vi "Diode Server.vi"() -> ()   [LabVIEW 2025]
uses:
  <vilib>/addons/_JKI Toolkits/State Machine/_JKI_lib_State_Machine.llb/Select State(s)_err__jki_lib_state_machine.vi
  <vilib>/addons/_JKI Toolkits/State Machine/_JKI_lib_State_Machine.llb/Periodic Trigger__ogtk__JKI-SM__jki_lib_state_machine.vi
  <instrlib>/ULx/ULx_LV.dll
  <instrlib>/Keithley 648X Series/Keithley 648X Series.lvlib
  <userlib>/_OpenG.lib/comparison/comparison.llb/openg_comparison__ogtk.lvlib
  <userlib>/_OpenG.lib/comparison/comparison.llb/Boolean Changed__ogtk.vi
panel:
  in  "Stimulate_LED":refnum<k21>
  in  "LED_Stimulate":bool
  in  "LED_Illuminate":bool
  out "D0 Measurement":dbl
  out "D1 Measurement":dbl
  in  "Illuminate_LED":refnum<k21>
  in  "MWIR PicoAmmeter":refnum<visa-resource-name>
  in  "SWIR Input":refnum<k21>="Dev0/Ai0"
  out "Diode Currents":waveform(dbl)[](graph)
  in  "Exit":bool
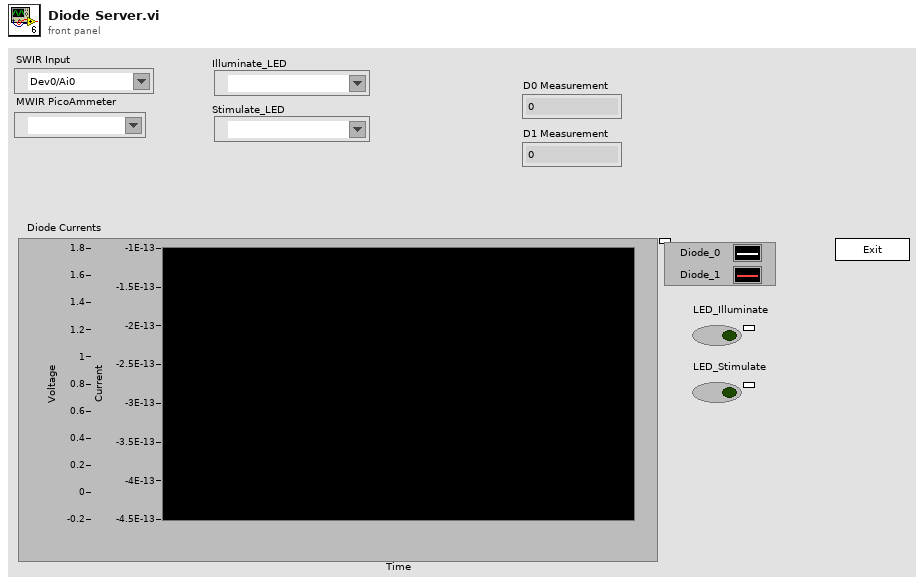
[diagram p1: front panel]
types:
  T1 = enum32{"Invalid", "Standard", "Closed", "Hidden", "Minimized", "Maximized"}
  T2 = enum32{"invalid app kind", "Development System", "Run Time System", "Student Edition", "Embedded LabVIEW", "Evaluation", "Custom"}
  T3 = cluster{"Core":cluster{"Current VI Reference":refnum<vi>, "Close Panel on Exit?":bool}, "Diode_Wfm":cluster{"Diode_Wfm":waveform(dbl)[]}, "Ulx SWIRMon":refnum<k24>, "ULx LED_Illum":refnum<k24>, "ULx LED_Stim":refnum<k24>, "PicoAmmeter VISA":refnum<visa-resource-name>}
  T4 = cluster{"Current VI Reference":refnum<vi>, "Close Panel on Exit?":bool}
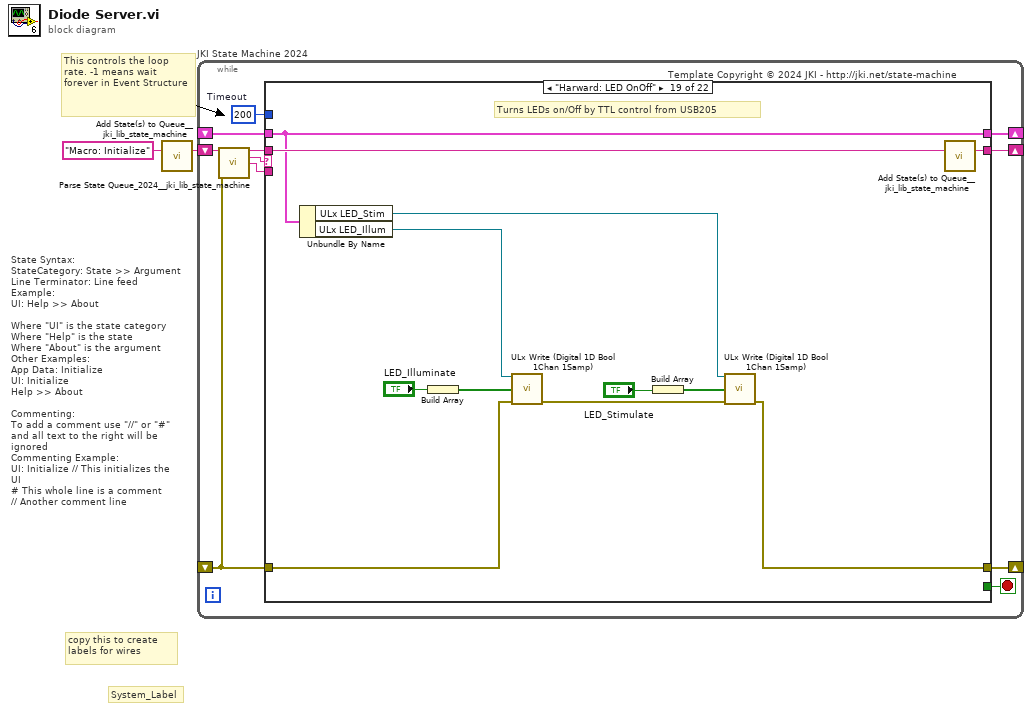
[diagram p0: block diagram]
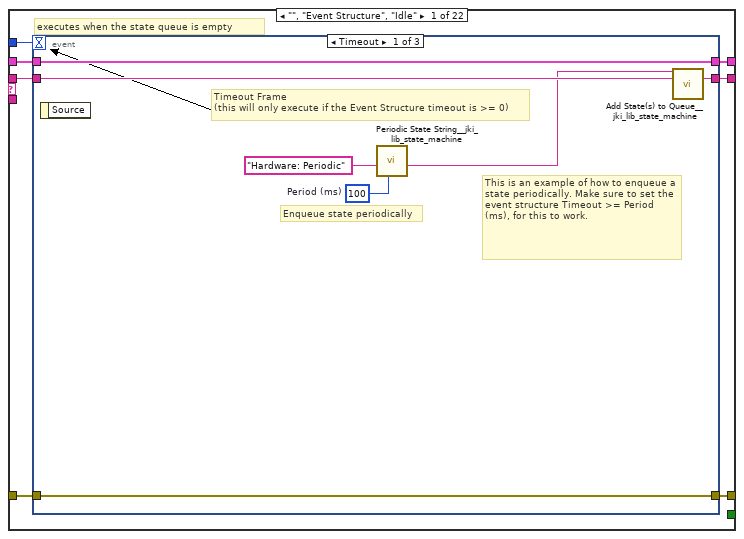
[diagram p2: hidden frame]
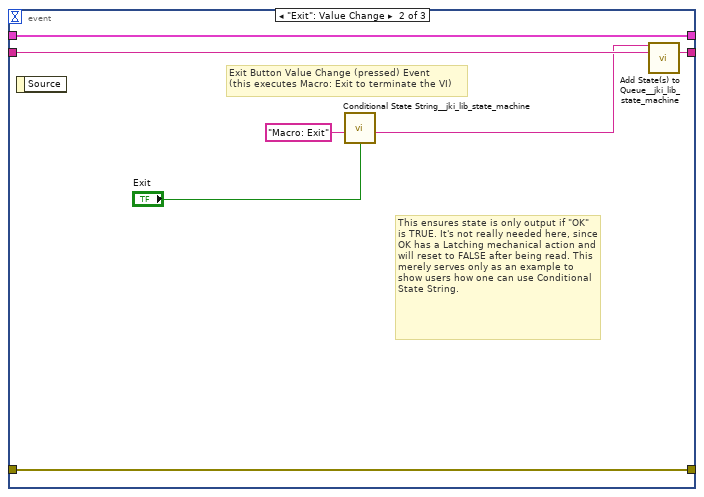
[diagram p3: hidden frame]
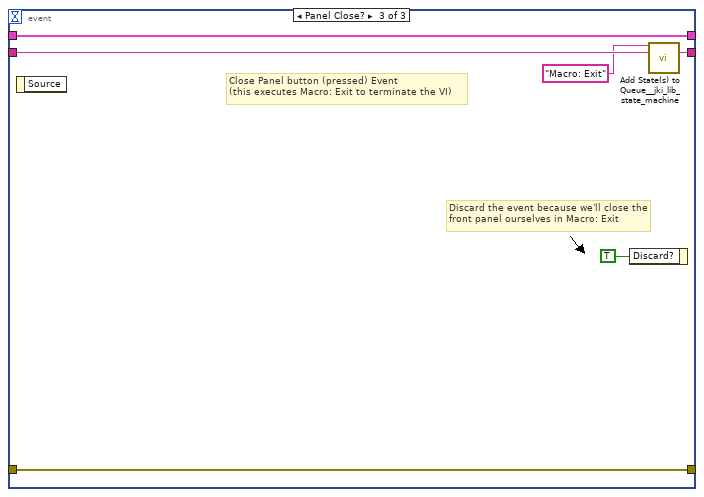
[diagram p4: hidden frame]
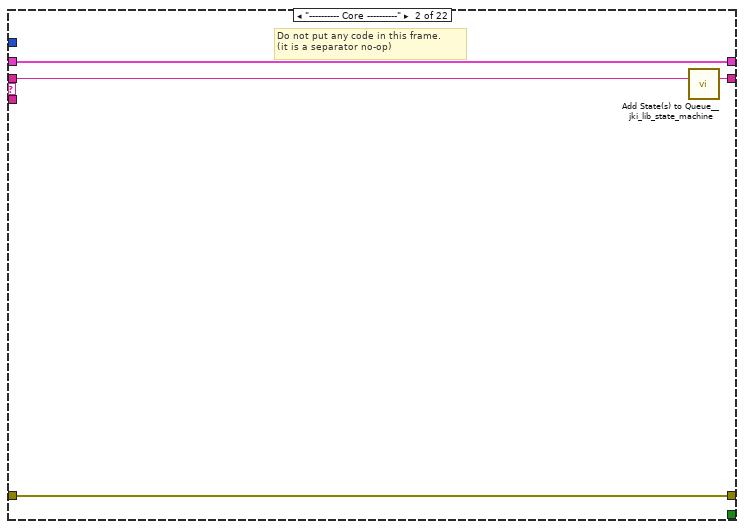
[diagram p5: hidden frame]
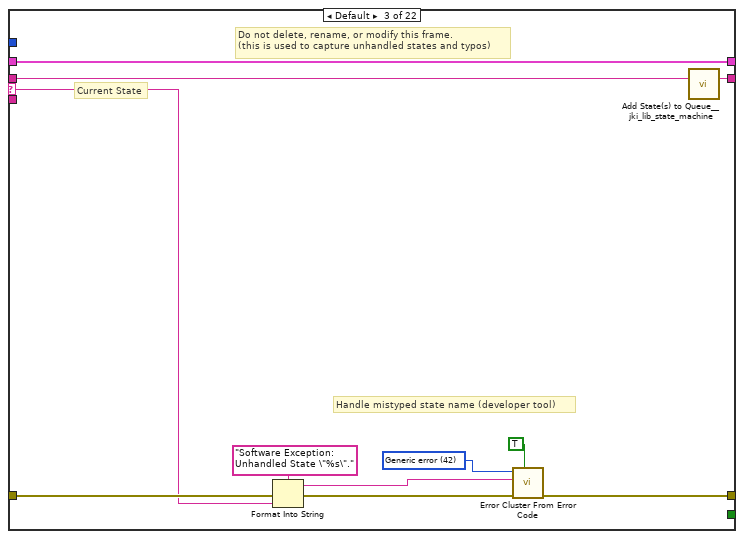
[diagram p6: hidden frame]
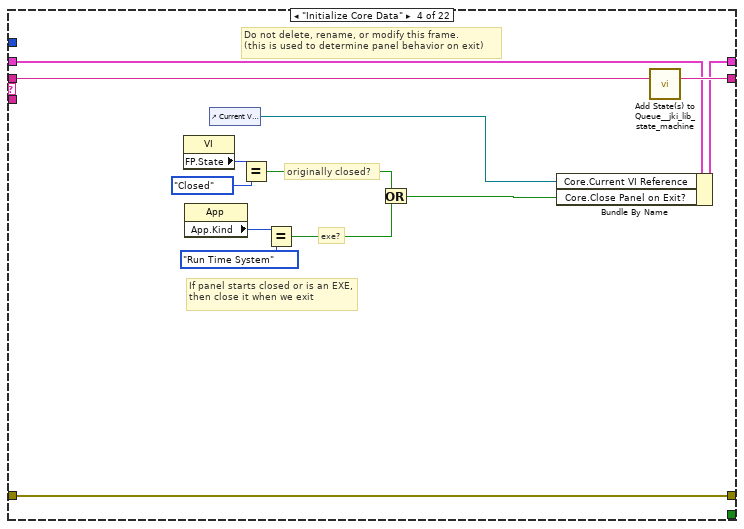
[diagram p7: hidden frame]
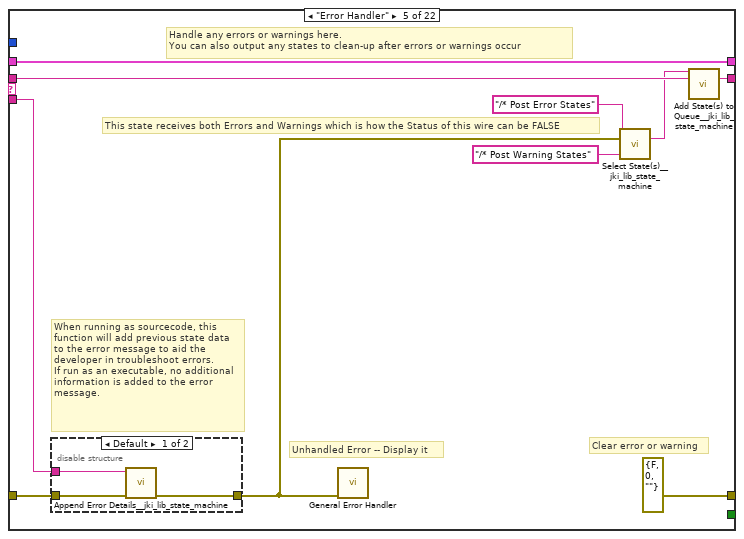
[diagram p8: hidden frame]
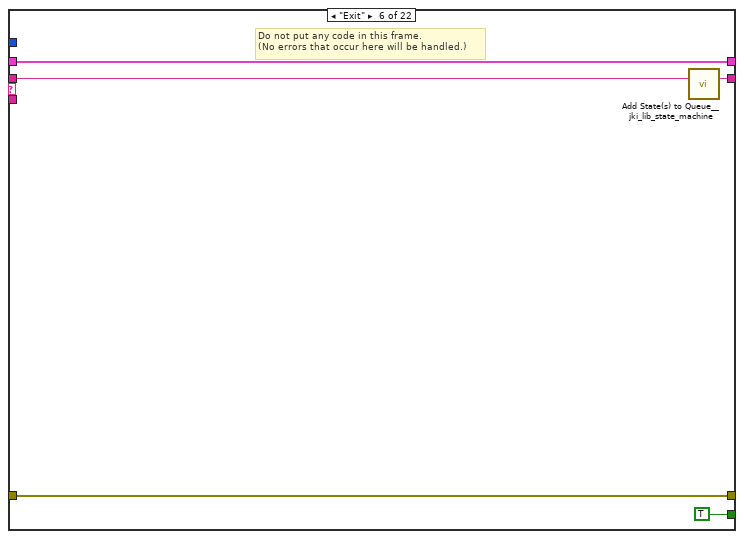
[diagram p10: hidden frame]
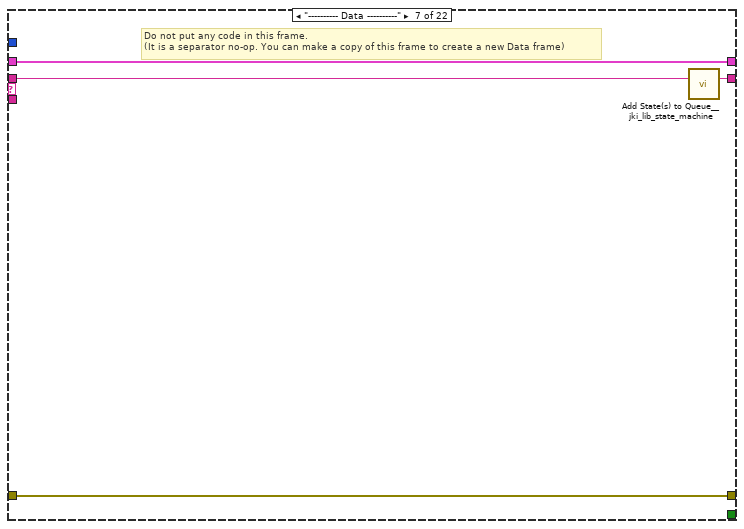
[diagram p11: hidden frame]
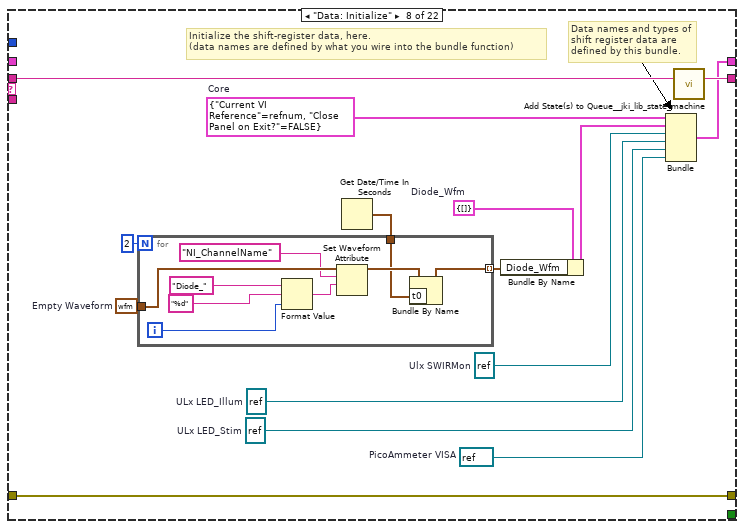
[diagram p12: hidden frame]
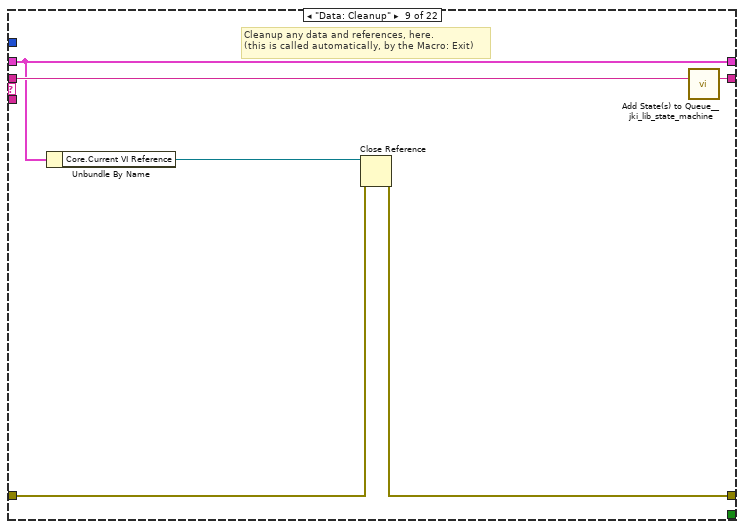
[diagram p13: hidden frame]
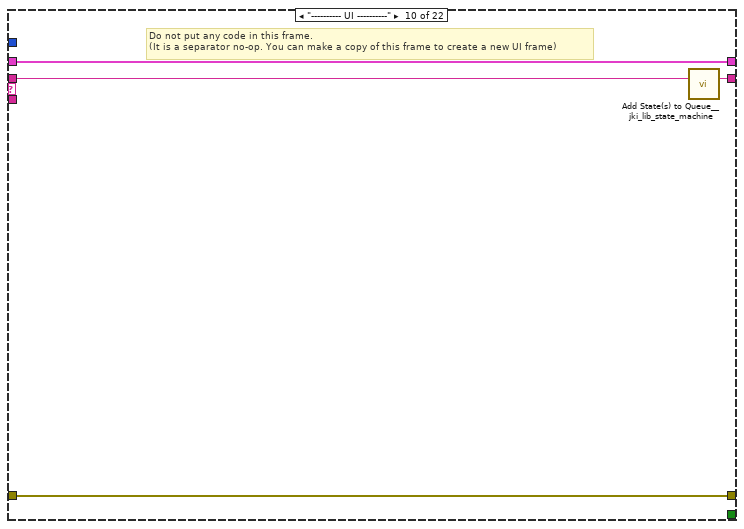
[diagram p14: hidden frame]
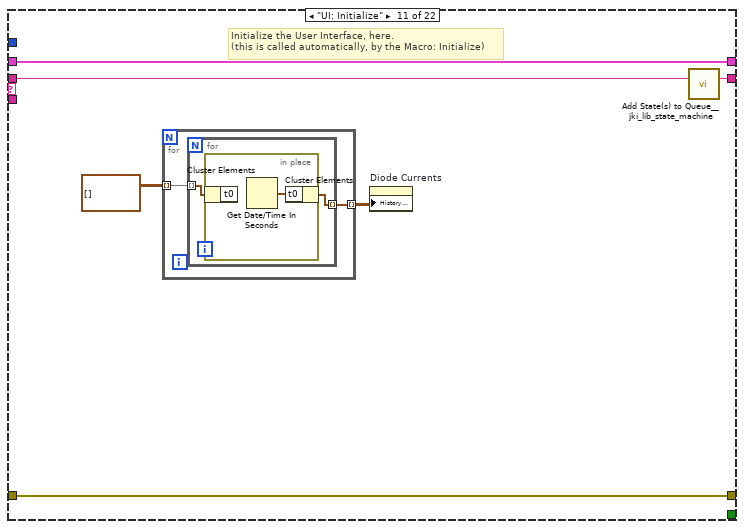
[diagram p15: hidden frame]
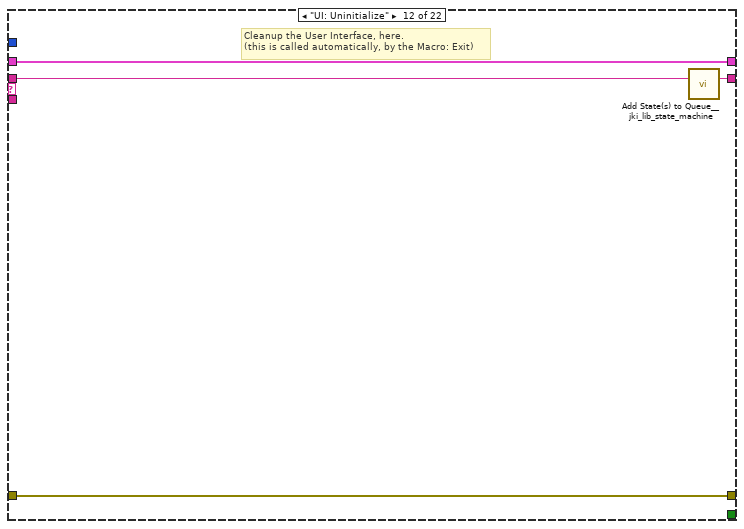
[diagram p16: hidden frame]
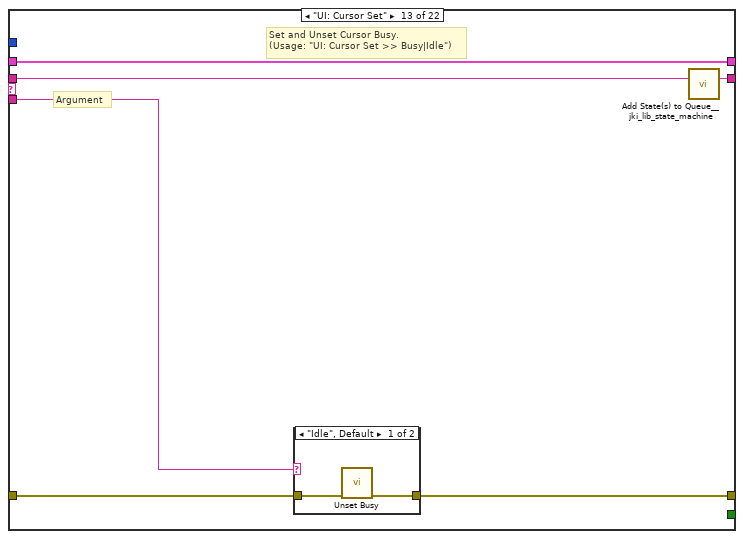
[diagram p17: hidden frame]
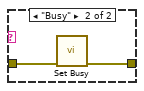
[diagram p18: hidden frame]
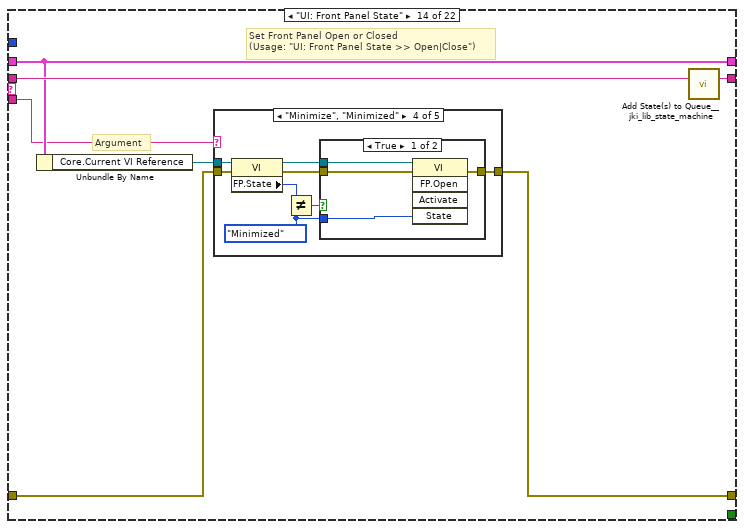
[diagram p19: hidden frame]
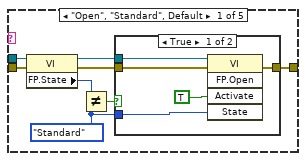
[diagram p20: hidden frame]
diagram:
  # "State Syntax:\nStateCategory: State >> Argument\nLine Terminator: Line feed\nExample:\nUI: Help >> About\n\nWhere \"UI\" is the state category\nWhere \"Help\" is the state\nWhere \"About\" is the argument\nOther Examples:\nApp Data: Initialize\nUI: Initialize\nHelp >> About\n\nCommenting:\nTo add a comment use \"//\" or \"#\" and all text to the right will be ignored\nCommenting Example:\nUI: Initialize // This initializes the UI\n# This whole line is a comment\n// Another comment line"
  # "copy this to create labels for wires"
  # "This controls the loop rate. -1 means wait forever in Event Structure"
  # "System_Label"
  n1 = call <vilib>:"Add State(s) to Queue__jki_lib_state_machine.vi"("State(s) in (\"\")"="Macro: Initialize") -> ("States Out"=w2:string)  [unwired: 14 in]
  n2 = while "JKI State Machine 2024" {
    shift-right: [w6] -> _
    shift-left: _ -> [w5]
    shift-right: [w9] -> _
    shift-left: _ -> [w3]
    shift-right: [w8] -> _
    shift-left: w2 -> [w10]
    stop <- w7 stop-if-true
    w4 = 200  # Timeout
    # "Template Copyright © 2024 JKI - http://jki.net/state-machine"
    n3 = call <vilib>:"Parse State Queue_2024__jki_lib_state_machine.vi"("State Queue"=w10, "Error In (no error)"=w3) -> ("Remaining States"=w12:string, "Current State"=w13:string, "Arguments"=w11:string)  [unwired: 11 in]
    n4 = case shown="\"Harward: LED OnOff\"" w13 {
      selector: w13 -> [_ _ w45 _ _ _ _ _ _ _ _ _ _ _ _ _ _ _ _ _ _ _]
      tunnel: w12 -> [w20 w44 w49 w68 w78 w87 w91 w106 w121 w125 w131 w140 w146 w157 w226 w231 w240 w244 w256 w275 w287 w305]
      tunnel: w11 -> [_ _ _ _ w73 _ _ _ _ _ _ _ w141 w151 _ _ _ _ _ _ _ _]
      tunnel: w5 -> [w18 w41 w47 w61 w75 w85 w88 _ w116 w122 w129 w138 w144 w153 w223 w228 w238 w241 w254 w273 w285 w298]
      tunnel: [w17 w42 w51 w65 errorcluster {"status"=FALSE, "code"=0, "source"=""} ("error out") w84 w89 w103 w117 w123 w128 w137 w142 w154 w224 w229 w235 w242 w247 w266 w281 w301] -> w9
      tunnel: w3 -> [w14 w42 w50 w65 w74 w84 w89 w103 w118 w123 w128 w137 w143 w155 w224 w229 w235 w242 w250 w271 w282 w302]
      tunnel: [w19 w43 w48 w67 w77 w86 w90 w105 w120 w124 w130 w139 w145 w156 w225 w230 w239 w243 w255 w274 w286 w304] -> w8
      tunnel: [_ _ _ _ _ TRUE _ _ _ _ _ _ _ _ _ _ _ _ _ _ _ _] -> w7
      tunnel: [w16 w41 w47 w66 w75 w85 w88 w104 w116 w122 w129 w138 w144 w153 w223 w228 w238 w241 w254 w268 w285 w296] -> w6
      tunnel: w4 -> [w15 _ _ _ _ _ _ _ _ _ _ _ _ _ _ _ _ _ _ _ _ _]
      frame "", "Event Structure", "Idle" {
        # "executes when the state queue is empty"
        n5 = event shown="[0] Timeout" {
          selector: _ -> [_ _ _]
          dyn-events: _ -> [_ _ _]
          timeout: w15 -> [_ _ _]
          tunnel: w20 -> [w27 w34 w40]
          tunnel: [w26 w33 w39] -> w19
          tunnel: w18 -> [w24 w31 w37]
          tunnel: [w25 w32 w38] -> w17
          tunnel: w14 -> [w25 w32 w38]
          tunnel: [w24 w31 w37] -> w16
          event Timeout {
            w21 = u32 100  # Period (ms)
            # "Enqueue state periodically"
            # "This is an example of how to enqueue a state periodically. Make sure to set the event structure Timeout >= Period (ms), for this to work."
            # "Timeout Frame\n(this will only execute if the Event Structure timeout is >= 0)"
            n6 = event-data() -> ()  [unwired: 1 in, 1 out]
            n7 = call <vilib>:"Periodic State String__jki_lib_state_machine.vi"("Period (ms)"=w21, "State"="Hardware: Periodic") -> ("State Out"=w23:string)  [unwired: 9 in]
            n8 = call <vilib>:"Add State(s) to Queue__jki_lib_state_machine.vi"("State(s) in Front (\"\")"=w23, "State(s) in (\"\")"=w27) -> ("States Out"=w26:string)  [unwired: 13 in]
          }
          event "Exit": Value Change {
            # "This ensures state is only output if \"OK\" is TRUE. It's not really needed here, since OK has a Latching mechanical action and will reset to FALSE after being read. This merely serves only as an example to show users how one can use Conditional State String."
            # "Exit Button Value Change (pressed) Event\n(this executes Macro: Exit to terminate the VI)"
            n9 = event-data() -> ()  [unwired: 1 in, 1 out]
            n10 = call <vilib>:"Conditional State String__jki_lib_state_machine.vi"("Do State(s)?"="Exit", "State"="Macro: Exit") -> ("State Out"=w28:string)  [unwired: 7 in]
            n11 = call <vilib>:"Add State(s) to Queue__jki_lib_state_machine.vi"("State(s) in Front (\"\")"=w28, "State(s) in (\"\")"=w34) -> ("States Out"=w33:string)  [unwired: 13 in]
          }
          event Panel Close? {
            # "Discard the event because we'll close the front panel ourselves in Macro: Exit"
            # "Close Panel button (pressed) Event\n(this executes Macro: Exit to terminate the VI)"
            n12 = event-data() -> ()  [unwired: 1 in, 1 out]
            n13 = event-data("Discard?"=TRUE) -> ()  [unwired: 1 in, 1 out]
            n14 = call <vilib>:"Add State(s) to Queue__jki_lib_state_machine.vi"("State(s) in Front (\"\")"="Macro: Exit", "State(s) in (\"\")"=w40) -> ("States Out"=w39:string)  [unwired: 13 in]
          }
        }
      }
      frame "---------- Core ----------" {
        # "Do not put any code in this frame.\n(it is a separator no-op)"
        n15 = call <vilib>:"Add State(s) to Queue__jki_lib_state_machine.vi"("State(s) in (\"\")"=w44) -> ("States Out"=w43:string)  [unwired: 14 in]
      }
      frame Default {
        w54 = 42 items=["No error", "Argument error", "Memory is full", "Out of zone", "End of file", "File already open", "Generic file I/O error", "File not found", "File permission error", "Disk is full", "Duplicate path", "Too many files open", "System feature not enabled", "Resource file not found", "Cannot add resource", "Resource not found", "Image not found", "Image memory error", "Pen does not exist", "Config type invalid", "Config token not found", "Config parse error", "Config memory error", "Bad external code format", "Bad external code offset", "External code not present", "Null window", "Destroy window error", "Null menu", "Print aborted", "Bad print record", "Print driver error", "Windows error during printing", "Memory error during printing", "Print dialog error", "Generic print error", "Invalid device refnum", "Device not found", "Device parameter error", "Device unit error", "Cannot open device", "Device call aborted", "Generic error", "Cancelled by user", "Object ID too low", "Object ID too high", "Object not in heap", "Unknown heap", "Unknown object (invalid DefProc)", "Unknown object (DefProc not in table)", "Message out of range", "Invalid (null) method", "Unknown message", "Manager call not supported", "Bad address", "Network operation in progress", "Network operation timed out", "Connection is busy", "Network attribute not supported", "Network error", "Address in use", "System out of memory", "Connection aborted", "Connection refused", "Not connected", "Already connected", "Connection closed", "Initialization error (interapplication manager)", "Bad occurrence", "Wait on unbound occurrence handler", "Occurrence queue overflow", "Datalog type conflict", "Unused", "Unrecognized type (interapplication manager)", "Memory corrupt", "Failed to make temporary DLL", "Old CIN version", "Drag socket not found", "Failed to load drop-object", "Failed to register OLE object", "Failed to release OLE object", "Format specifier type mismatch", "Unknown format specifier", "Too few format specifiers", "Too many format specifiers", "Scan failed", "Newer CIN version", "Error converting to variant", "Runtime menu error", "Password tampered", "Variant attribute not found", "Incompatible variant data type", "Event data is not available", "Event Store is not present", "Occurrence is not found", "Event Queue is not created", "Event info is not available", "Refnum passed is NULL", "Error retrieving Class GUID", "Error retrieving CoClass GUID", "Error retrieving TypeLib GUID.", "Bad built application magic bytes.", "Specific driver is different from the specific driver associated with the Logical Name.", "There is no session opened to the class driver.", "Max Error", "MAX - Error with config objects", "MAX - Error loading configuration", "MAX - Group not supported"]
        # "Current State"
        # "Do not delete, rename, or modify this frame.\n(this is used to capture unhandled states and typos)"
        # "Handle mistyped state name (developer tool)"
        n16 = Format Into String(format string="Software Exception: Unhandled State \"%s\"." ("message"), error in=w50, w45) -> (resulting string=w53:string, error out=w52:errorcluster)  [unwired: 1 in]
        n17 = call <vilib>:"Error Cluster From Error Code.vi"("show call chain? (False)"=TRUE, "error in (no error)"=w52, "error message (\"\")"=w53, "error code (0)"=w54) -> ("error out"=w51:errorcluster)  [unwired: 5 in]
        n18 = call <vilib>:"Add State(s) to Queue__jki_lib_state_machine.vi"("State(s) in (\"\")"=w49) -> ("States Out"=w48:string)  [unwired: 14 in]
      }
      frame "Initialize Core Data" {
        # "Do not delete, rename, or modify this frame.\n(this is used to determine panel behavior on exit)"
        # "originally closed?"
        # "exe?"
        # "If panel starts closed or is an EXE, then close it when we exit"
        n19 = property class="VI"() -> ("FP.State"=w58:T1)  [unwired: 2 in, 2 out]
        n20 = property class="App"() -> ("App.Kind"=w64:T2)  [unwired: 2 in, 2 out]
        n21 = control-ref of="Current VI Reference"() -> (w59:refnum<vi>)
        n22 = Equal?(x=w58, y=T1."Closed" ("Front Panel Window:State")) -> (x = y?=w56:bool)
        n23 = Equal?(x=w64, y=T2."Run Time System" ("Application:Kind")) -> (x = y?=w62:bool)
        n24 = Or(x=w56, y=w62) -> (x .or. y?=w60:bool)
        n25 = Bundle By Name(cluster=w61, "Core.Current VI Reference"=w59, "Core.Close Panel on Exit?"=w60) -> (w66:T3)
        n26 = call <vilib>:"Add State(s) to Queue__jki_lib_state_machine.vi"("State(s) in (\"\")"=w68) -> ("States Out"=w67:string)  [unwired: 14 in]
      }
      frame "Error Handler" {
        # "When running as sourcecode, this function will add previous state data to the error message to aid the developer in troubleshoot errors.\nIf run as an executable, no additional information is added to the error message."
        # "This state receives both Errors and Warnings which is how the Status of this wire can be FALSE"
        # "Unhandled Error -- Display it"
        # "Handle any errors or warnings here.\nYou can also output any states to clean-up after errors or warnings occur"
        # "Clear error or warning"
        n27 = disable-structure shown="Default" {
          disable-tunnel: w74 -> [w81 w82]
          disable-tunnel: w73 -> [w80 _]
          disable-tunnel: [w79 w82] -> w72
          frame condition #0 (active) {
            n28 = call <vilib>:"Append Error Details__jki_lib_state_machine.vi"("error in (no error)"=w81, "Previous State and Argument(s)"=w80) -> ("error out"=w79:errorcluster)  [unwired: 9 in]
          }
          frame condition #1 {
          }
        }
        n29 = call <vilib>:"General Error Handler.vi"("error in (no error)"=w72) -> ()  [unwired: 10 in, 5 out]
        n30 = call-poly <vilib>:"Select State(s)__jki_lib_state_machine.vi"("State(s) if True (\"\")"="/* Post Error States", "Select"=w72, "State(s) if False (\"\")"="/* Post Warning States") -> ("States Out"=w70:string)  [unwired: 12 in]
        n31 = call <vilib>:"Add State(s) to Queue__jki_lib_state_machine.vi"("State(s) in Front (\"\")"=w70, "State(s) in (\"\")"=w78) -> ("States Out"=w77:string)  [unwired: 13 in]
      }
      frame "Exit" {
        # "Do not put any code in this frame.\n(No errors that occur here will be handled.)"
        n32 = call <vilib>:"Add State(s) to Queue__jki_lib_state_machine.vi"("State(s) in (\"\")"=w87) -> ("States Out"=w86:string)  [unwired: 14 in]
      }
      frame "---------- Data ----------" {
        # "Do not put any code in this frame.\n(It is a separator no-op. You can make a copy of this frame to create a new Data frame)"
        n33 = call <vilib>:"Add State(s) to Queue__jki_lib_state_machine.vi"("State(s) in (\"\")"=w91) -> ("States Out"=w90:string)  [unwired: 14 in]
      }
      frame "Data: Initialize" {
        w92 = refnum<k24> refnum  # ULx LED_Stim
        w100 = cluster{"Diode_Wfm":waveform(dbl)[]} {"Diode_Wfm"=[]}  # Diode_Wfm
        w94 = refnum<visa-resource-name> refnum  # PicoAmmeter VISA
        w93 = refnum<k24> refnum  # ULx LED_Illum
        w96 = refnum<k24> refnum  # Ulx SWIRMon
        w98 = waveform(dbl) {"t0"=timestamp(0 s since 1904-01-01), "dt"=1.0, "Y"=[]}  # Empty Waveform
        w102 = T4 {"Current VI Reference"=refnum, "Close Panel on Exit?"=FALSE}  # Core
        # "Data names and types of shift register data are defined by this bundle."
        # "Initialize the shift-register data, here.\n(data names are defined by what you wire into the bundle function)"
        n34 = Get Date/Time In Seconds() -> (seconds since 1Jan1904=w95:timestamp)
        n35 = for {
          N: 2 -> [_]
          tunnel: w98 -> [w112]
          tunnel: [w108] -> w101 mode=indexing
          tunnel: w95 -> [w107]
          i -> [w109]
          n36 = Format Value(string ("")="Diode_", format string="%d", value (0)=w109) -> (output string=w114:string)
          n37 = Set Waveform Attribute(5:w114, 6:"NI_ChannelName" ("name"), 7:w112) -> (3:w111:waveform(dbl))  [unwired: 1 in, 2 out]
          n38 = Bundle By Name(cluster=w111, "t0"=w107) -> (w108:waveform(dbl))
        }
        n39 = Bundle By Name(cluster=w100, "Diode_Wfm"=w101) -> (w97:cluster{"Diode_Wfm":waveform(dbl)[]})
        n40 = Bundle("Core"=w102, "Diode_Wfm"=w97, "Ulx SWIRMon"=w96, "ULx LED_Illum"=w93, "ULx LED_Stim"=w92, "PicoAmmeter VISA"=w94) -> (w104:T3)  [unwired: 1 in]
        n41 = call <vilib>:"Add State(s) to Queue__jki_lib_state_machine.vi"("State(s) in (\"\")"=w106) -> ("States Out"=w105:string)  [unwired: 14 in]
      }
      frame "Data: Cleanup" {
        # "Cleanup any data and references, here.\n(this is called automatically, by the Macro: Exit)"
        n42 = Unbundle By Name(w116) -> ("Core.Current VI Reference"=w119:refnum<vi>)
        n43 = Close Reference(reference=w119, error in (no error)=w118) -> (error out=w117:errorcluster)
        n44 = call <vilib>:"Add State(s) to Queue__jki_lib_state_machine.vi"("State(s) in (\"\")"=w121) -> ("States Out"=w120:string)  [unwired: 14 in]
      }
      frame "---------- UI ----------" {
        # "Do not put any code in this frame.\n(It is a separator no-op. You can make a copy of this frame to create a new UI frame)"
        n45 = call <vilib>:"Add State(s) to Queue__jki_lib_state_machine.vi"("State(s) in (\"\")"=w125) -> ("States Out"=w124:string)  [unwired: 14 in]
      }
      frame "UI: Initialize" {
        # "Initialize the User Interface, here.\n(this is called automatically, by the Macro: Initialize)"
        n46 = for {
          tunnel: waveform(dbl)[][] [] ("History Data") -> [w133] mode=indexing
          tunnel: [w132] -> w126 mode=indexing
          n47 = for {
            tunnel: w133 -> [w135] mode=indexing
            tunnel: [w134] -> w132 mode=indexing
            n48 = in-place {
              n49 = in-place-cluster #1(w135) -> ()  [unwired: 1 out]
              n50 = Get Date/Time In Seconds() -> (seconds since 1Jan1904=w136:timestamp)
              n51 = in-place-cluster #1("t0"=w136) -> (w134:waveform(dbl))
            }
          }
        }
        n52 = property on="Diode Currents" class="WFChart (strict)"("History Data"=w126) -> ()  [unwired: 2 in, 2 out]
        n53 = call <vilib>:"Add State(s) to Queue__jki_lib_state_machine.vi"("State(s) in (\"\")"=w131) -> ("States Out"=w130:string)  [unwired: 14 in]
      }
      frame "UI: Uninitialize" {
        # "Cleanup the User Interface, here.\n(this is called automatically, by the Macro: Exit)"
        n54 = call <vilib>:"Add State(s) to Queue__jki_lib_state_machine.vi"("State(s) in (\"\")"=w140) -> ("States Out"=w139:string)  [unwired: 14 in]
      }
      frame "UI: Cursor Set" {
        # "Argument"
        # "Set and Unset Cursor Busy.\n(Usage: \"UI: Cursor Set >> Busy|Idle\")"
        n55 = case shown="\"Idle\", Default" w141 {
          tunnel: w143 -> [w148 w150]
          tunnel: [w147 w149] -> w142
          frame "Idle", Default {
            n56 = call <vilib>:"Unset Busy.vi"("error in (no error)"=w148) -> ("error out"=w147:errorcluster)  [unwired: 10 in]
          }
          frame "Busy" {
            n57 = call <vilib>:"Set Busy.vi"("error in (no error)"=w150) -> ("error out"=w149:errorcluster)  [unwired: 9 in, 1 out]
          }
        }
        n58 = call <vilib>:"Add State(s) to Queue__jki_lib_state_machine.vi"("State(s) in (\"\")"=w146) -> ("States Out"=w145:string)  [unwired: 14 in]
      }
      frame "UI: Front Panel State" {
        # "Argument"
        # "Set Front Panel Open or Closed\n(Usage: \"UI: Front Panel State >> Open|Close\")"
        n59 = Unbundle By Name(w153) -> ("Core.Current VI Reference"=w152:refnum<vi>)
        n60 = case shown="\"Minimize\", \"Minimized\"" w151 {
          tunnel: w155 -> [w163 w178 w189 w202 w215]
          tunnel: [w165 w179 w191 w204 w217] -> w154
          tunnel: w152 -> [w164 w176 w190 w203 w216]
          frame "Open", "Standard", Default {
            w158 = T1."Standard" ("State")
            n61 = property class="VI"(reference=w164, error in=w163) -> (reference out=w161:refnum<vi>, error out=w162:errorcluster, "FP.State"=w160:T1)
            n62 = Not Equal?(x=w160, y=w158) -> (x != y?=w159:bool)
            n63 = case shown="True" w159 {
              tunnel: [w169 w171] -> w165
              tunnel: w162 -> [w168 w171]
              tunnel: w161 -> [w167 _]
              tunnel: w158 -> [w166 _]
              frame True {
                n64 = invoke class="VI" method="FP.Open"(reference=w167, error in=w168, "Activate"=TRUE, "State"=w166) -> (error out=w169:errorcluster)  [unwired: 1 in, 4 out]
              }
              frame False {
              }
            }
          }
          frame "Close", "Closed" {
            n65 = property class="VI"(reference=w176, error in=w178) -> (reference out=w175:refnum<vi>, error out=w177:errorcluster, "FP.State"=w173:T1)
            n66 = Not Equal?(x=w173, y=T1."Closed" ("Front Panel Window:State")) -> (x != y?=w172:bool)
            n67 = case shown="True" w172 {
              tunnel: [w180 w183] -> w179
              tunnel: w177 -> [w180 w182]
              tunnel: w175 -> [_ w181]
              frame False {
              }
              frame True {
                n68 = invoke class="VI" method="FP.Close"(reference=w181, error in=w182) -> (error out=w183:errorcluster)  [unwired: 1 in, 2 out]
              }
            }
          }
          frame "Hidden", "Hide" {
            w184 = T1."Hidden" ("State")
            n69 = property class="VI"(reference=w190, error in=w189) -> (reference out=w187:refnum<vi>, error out=w188:errorcluster, "FP.State"=w186:T1)
            n70 = Not Equal?(x=w186, y=w184) -> (x != y?=w185:bool)
            n71 = case shown="True" w185 {
              tunnel: [w195 w196] -> w191
              tunnel: w188 -> [w194 w196]
              tunnel: w187 -> [w193 _]
              tunnel: w184 -> [w192 _]
              frame True {
                n72 = invoke class="VI" method="FP.Open"(reference=w193, error in=w194, "State"=w192) -> (error out=w195:errorcluster)  [unwired: 2 in, 4 out]
              }
              frame False {
              }
            }
          }
          frame "Minimize", "Minimized" {
            w197 = T1."Minimized" ("State")
            n73 = property class="VI"(reference=w203, error in=w202) -> (reference out=w200:refnum<vi>, error out=w201:errorcluster, "FP.State"=w199:T1)
            n74 = Not Equal?(x=w199, y=w197) -> (x != y?=w198:bool)
            n75 = case shown="True" w198 {
              tunnel: [w208 w209] -> w204
              tunnel: w201 -> [w207 w209]
              tunnel: w200 -> [w206 _]
              tunnel: w197 -> [w205 _]
              frame True {
                n76 = invoke class="VI" method="FP.Open"(reference=w206, error in=w207, "State"=w205) -> (error out=w208:errorcluster)  [unwired: 2 in, 4 out]
              }
              frame False {
              }
            }
          }
          frame "Maximize", "Maximized" {
            w210 = T1."Maximized" ("State")
            n77 = property class="VI"(reference=w216, error in=w215) -> (reference out=w213:refnum<vi>, error out=w214:errorcluster, "FP.State"=w212:T1)
            n78 = Not Equal?(x=w212, y=w210) -> (x != y?=w211:bool)
            n79 = case shown="True" w211 {
              tunnel: [w221 w222] -> w217
              tunnel: w214 -> [w220 w222]
              tunnel: w213 -> [w219 _]
              tunnel: w210 -> [w218 _]
              frame True {
                n80 = invoke class="VI" method="FP.Open"(reference=w219, error in=w220, "State"=w218) -> (error out=w221:errorcluster)  [unwired: 2 in, 4 out]
              }
              frame False {
              }
            }
          }
        }
        n81 = call <vilib>:"Add State(s) to Queue__jki_lib_state_machine.vi"("State(s) in (\"\")"=w157) -> ("States Out"=w156:string)  [unwired: 14 in]
      }
      frame "---------- Macro ----------" {
        # "Do not put any code in this frame.\n(It is a separator no-op. You can make a copy of this frame to create a new Macro frame)"
        n82 = call <vilib>:"Add State(s) to Queue__jki_lib_state_machine.vi"("State(s) in (\"\")"=w226) -> ("States Out"=w225:string)  [unwired: 14 in]
      }
      frame "Macro: Initialize" {
        w227 = "Data: Initialize\nInitialize Core Data\nUI: Initialize\nUI: Front Panel State >> Open\nHardware: Initialize"  # Data: Initialize Initialize Core Data UI: Initialize UI: Front Panel State >> Open Hardware: Initialize
        # "Initialization Macro\n(This is called once, when the VI starts)"
        n83 = call <vilib>:"Add State(s) to Queue__jki_lib_state_machine.vi"("State(s) in Front (\"\")"=w227, "State(s) in (\"\")"=w231) -> ("States Out"=w230:string)  [unwired: 13 in]
      }
      frame "Macro: Exit" {
        # "Exit Macro\n(This is called once, when the VI exits)"
        n84 = Unbundle By Name(w238) -> ("Core.Close Panel on Exit?"=w233:bool)
        n85 = call <vilib>:"Conditional State String__jki_lib_state_machine.vi"("Do State(s)?"=w233, "State"="UI: Front Panel State >> Close") -> ("State Out"=w232:string)  [unwired: 7 in]
        n86 = call <vilib>:"Add State(s) to Queue__jki_lib_state_machine.vi"("State(s) in (\"\")"=w232, "State(s) at Back (\"\")"="Hardware: Cleanup\nUI: Uninitialize\nData: Cleanup\nExit") -> ("States Out"=w236:string)  [unwired: 13 in]
        n87 = call <vilib>:"Add State(s) to Queue__jki_lib_state_machine.vi"("State(s) in Front (\"\")"=w236, "State(s) in (\"\")"=w240) -> ("States Out"=w239:string)  [unwired: 13 in]
      }
      frame "---------- Hardware ----------" {
        # "Template Separator\n(You can make a copy of, or modify, this frame)"
        n88 = call <vilib>:"Add State(s) to Queue__jki_lib_state_machine.vi"("State(s) in (\"\")"=w244) -> ("States Out"=w243:string)  [unwired: 14 in]
      }
      frame "Harward: LED OnOff" {
        # "Turns LEDs on/Off by TTL control from USB205"
        n89 = Unbundle By Name(w254) -> ("ULx LED_Stim"=w252:refnum<k24>, "ULx LED_Illum"=w253:refnum<k24>)
        n90 = Build Array("LED_Illuminate") -> (w248:bool[])
        n91 = call <instrlib>:"ULx Write (Digital 1D Bool 1Chan 1Samp).vi"("task in"=w253, "data"=w248, "error in"=w250) -> ("error out"=w251:errorcluster)  [unwired: 10 in, 2 out]
        n92 = Build Array("LED_Stimulate") -> (w245:bool[])
        n93 = call <instrlib>:"ULx Write (Digital 1D Bool 1Chan 1Samp).vi"("task in"=w252, "data"=w245, "error in"=w251) -> ("error out"=w247:errorcluster)  [unwired: 10 in, 2 out]
        n94 = call <vilib>:"Add State(s) to Queue__jki_lib_state_machine.vi"("State(s) in (\"\")"=w256) -> ("States Out"=w255:string)  [unwired: 14 in]
      }
      frame "Hardware: Initialize" {
        # "Analogue in for SWIR"
        # "Initialise Hardware"
        n95 = call <instrlib>:"ULx Create Channel (AI-Voltage-Basic).vi"("maximum value"=10.0, "minimum value"=0.0, "physical channels"="SWIR Input", "error in"=w271) -> ("task out"=w267:refnum<k24>, "error out"=w264:errorcluster)  [unwired: 10 in]
        n96 = call <instrlib>:"ULx Create Channel (DO-Digital Output).vi"("lines"="Illuminate_LED", "error in"=w264) -> ("task out"=w263:refnum<k24>, "error out"=w260:errorcluster)  [unwired: 12 in]
        n97 = call <instrlib>:"ULx Create Channel (DO-Digital Output).vi"("lines"="Stimulate_LED", "error in"=w260) -> ("task out"=w257:refnum<k24>, "error out"=w259:errorcluster)  [unwired: 12 in]
        n98 = call <instrlib>:"Initialize.vi"("error in (no error)"=w259, "VISA resource name"="MWIR PicoAmmeter") -> ("error out"=w266:errorcluster, "VISA resource name out"=w262:refnum<visa-resource-name>)  [unwired: 8 in]
        n99 = Bundle By Name(cluster=w273, "Ulx SWIRMon"=w267, "ULx LED_Illum"=w263, "ULx LED_Stim"=w257, "PicoAmmeter VISA"=w262) -> (w268:T3)
        n100 = call <vilib>:"Add State(s) to Queue__jki_lib_state_machine.vi"("State(s) in (\"\")"=w275) -> ("States Out"=w274:string)  [unwired: 14 in]
      }
      frame "Hardware: Cleanup" {
        # "Close ULx channels\nClose PicoAmmeter"
        n101 = Unbundle By Name(w285) -> ("PicoAmmeter VISA"=w280:refnum<visa-resource-name>, "ULx LED_Stim"=w278:refnum<k24>, "ULx LED_Illum"=w279:refnum<k24>, "Ulx SWIRMon"=w284:refnum<k24>)
        n102 = call <instrlib>:"ULx Clear Task.vi"("task in"=w284, "error in"=w282) -> ("error out"=w283:errorcluster)  [unwired: 13 in]
        n103 = call <instrlib>:"ULx Clear Task.vi"("task in"=w279, "error in"=w283) -> ("error out"=w277:errorcluster)  [unwired: 13 in]
        n104 = call <instrlib>:"ULx Clear Task.vi"("task in"=w278, "error in"=w277) -> ("error out"=w276:errorcluster)  [unwired: 13 in]
        n105 = call <instrlib>:"Close.vi"("error in (no error)"=w276, "VISA resource name"=w280) -> ("error out"=w281:errorcluster)  [unwired: 9 in]
        n106 = call <vilib>:"Add State(s) to Queue__jki_lib_state_machine.vi"("State(s) in (\"\")"=w287) -> ("States Out"=w286:string)  [unwired: 14 in]
      }
      frame "Hardware: Periodic" {
        # "Read and Update Graph\nTalks to USB205 and Keithley Picoammeter"
        n107 = Unbundle By Name(w298) -> ("PicoAmmeter VISA"=w299:refnum<visa-resource-name>, "Ulx SWIRMon"=w303:refnum<k24>)
        n108 = call <instrlib>:"ULx Read (Analog DBL 1Chan 1Samp).vi"("task in"=w303, "error in"=w302) -> ("data"=w295:dbl, "error out"=w300:errorcluster)  [unwired: 11 in, 1 out]
        "D0 Measurement" <- w295
        n109 = call <instrlib>:"Measure Current.vi"("VISA resource name"=w299, "error in (no error)"=w300) -> ("Measurement"=w297:dbl, "error out"=w301:errorcluster)  [unwired: 11 in, 1 out]
        "D1 Measurement" <- w297
        n110 = in-place {
          in-place-border: w297 -> [w310]
          in-place-border: w295 -> [w309]
          n111 = in-place-cluster #2(w298) -> ("Diode_Wfm.Diode_Wfm"=w311:waveform(dbl)[])
          n112 = Build Array(w309, w310) -> (w308:dbl[])
          n113 = Get Date/Time In Seconds() -> (seconds since 1Jan1904=w307:timestamp)
          n114 = for {
            tunnel: w311 -> [w315] mode=indexing
            tunnel: w308 -> [w316] mode=indexing
            tunnel: w307 -> [w313]
            tunnel: [w312] -> w306 mode=indexing
            n115 = Build Array(w316) -> (w314:dbl[])
            n116 = Bundle By Name(cluster=w315, "t0"=w313, "Y"=w314) -> (w312:waveform(dbl))
          }
          "Diode Currents" <- w306
          n117 = in-place-cluster #2("Diode_Wfm.Diode_Wfm"=w306) -> (w296:T3)
        }
        n118 = local read "LED_Illuminate"() -> (w294:bool)
        n119 = local read "LED_Stimulate"() -> (w293:bool)
        n120 = call-poly <userlib>:"Data Changed__ogtk.vi"("Boolean"=w293) -> ("Changed"=w291:bool)
        n121 = call-poly <userlib>:"Data Changed__ogtk.vi"("Boolean"=w294) -> ("Changed"=w292:bool)
        n122 = Or(x=w292, y=w291) -> (x .or. y?=w290:bool)
        n123 = call <vilib>:"Conditional State String__jki_lib_state_machine.vi"("Do State(s)?"=w290, "State"="Harward: LED OnOff") -> ("State Out"=w289:string)  [unwired: 7 in]
        n124 = call <vilib>:"Add State(s) to Queue__jki_lib_state_machine.vi"("State(s) in (\"\")"=w305, "State(s) at Back (\"\")"=w289) -> ("States Out"=w304:string)  [unwired: 13 in]
      }
    }
  }
